vi "MojoTest.vi"() -> ()   [LabVIEW 2018]
panel:
  in  "Port":refnum<visa-resource-name>
  in  "LED":u8
  in  "stop":bool
  out "Waveform Graph":i32[](graph)
  out "XY Graph":cluster{i32[], "Data Out":i32[]}(graph)
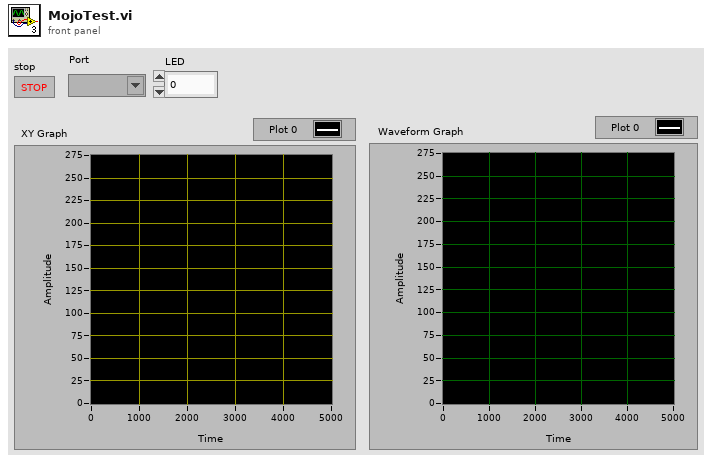
[diagram p1: front panel]
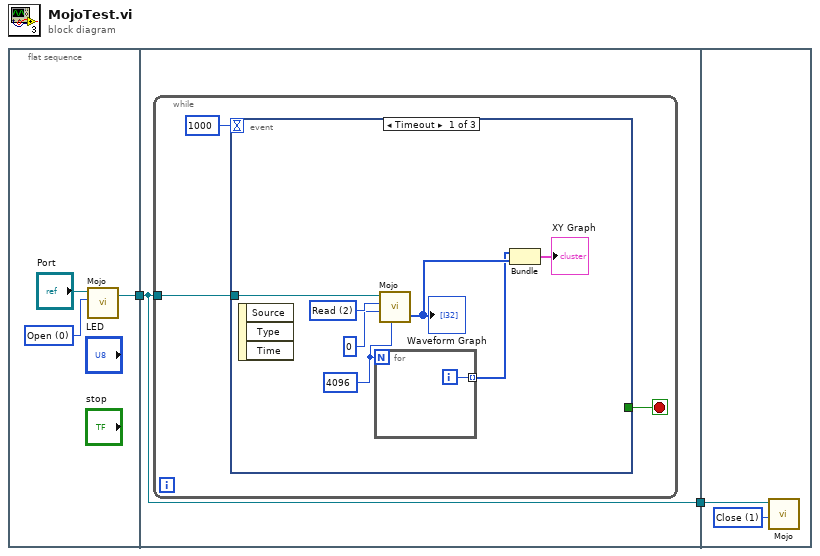
[diagram p0: block diagram]
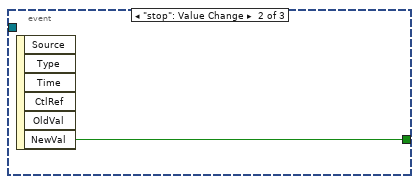
[diagram p2: hidden frame]
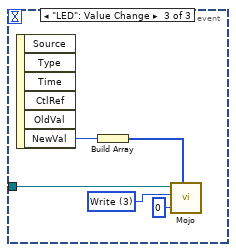
[diagram p3: hidden frame]
diagram:
  n1 = flat-sequence {
    tunnel: [w3] -> w2
    tunnel: w2 -> [w6]
    tunnel: [w6] -> w1
    tunnel: w1 -> [w25]
    frame #0 {
      w4 = u8 0 items=["Open", "Close", "Read", "Write"] ("Mode")
      n2 = call "Mojo.vi"("Mode"=w4, "Port In"="Port") -> ("Port Out"=w3:refnum<visa-resource-name>)  [unwired: 4 in, 1 out]
    }
    frame #1 {
      n3 = while {
        tunnel: w6 -> [w8]
        stop <- w9 stop-if-true
        n4 = event shown="[0] Timeout" {
          selector: _ -> [_ _ _]
          dyn-events: _ -> [_ _ _]
          timeout: 1000 -> [_ _ _]
          tunnel: [_ w18 _] -> w9
          tunnel: w8 -> [w16 _ w21]
          event Timeout {
            w12 = i16 4096 ("Length")
            w15 = u8 2 items=["Open", "Close", "Read", "Write"] ("Mode")
            n5 = event-data() -> ()  [unwired: 1 in, 3 out]
            n6 = for {
              N: w12 -> [_]
              tunnel: [w17] -> w11 mode=indexing
              i -> [w17]
            }
            n7 = call "Mojo.vi"("Length"=w12, "Address"=u32 0, "Mode"=w15, "Port In"=w16) -> ("Data Out"=w13:i32[])  [unwired: 2 in, 1 out]
            "Waveform Graph" <- w13
            n8 = Bundle(w11, "Data Out"=w13) -> (→"XY Graph":cluster{i32[], "Data Out":i32[]})  [unwired: 1 in]
          }
          event "stop": Value Change {
            n9 = event-data() -> ("NewVal"=w18:bool)  [unwired: 1 in, 5 out]
          }
          event "LED": Value Change {
            w20 = u8 3 items=["Open", "Close", "Read", "Write"] ("Mode")
            n10 = event-data() -> ("NewVal"=w23:u8)  [unwired: 1 in, 5 out]
            n11 = Build Array(w23) -> (w22:u8[])
            n12 = call "Mojo.vi"("Data In"=w22, "Address"=u32 0, "Mode"=w20, "Port In"=w21) -> ()  [unwired: 2 in, 2 out]
          }
        }
      }
    }
    frame #2 {
      w24 = u8 1 items=["Open", "Close", "Read", "Write"] ("Mode")
      n13 = call "Mojo.vi"("Mode"=w24, "Port In"=w25) -> ()  [unwired: 4 in, 2 out]
    }
  }
